vi "2_2_PatchCore_Inference(Camera).vi"() -> ()   [LabVIEW 2024]
uses:
  <vilib>/Ngene/DeepLTK Anomaly Detection Addon/DeepLTK_Anomaly_Detection_Addon/API/Controls/NN_Paths.ctl
  <vilib>/Ngene/Deep Learning Toolkit/Toolkit/NN_Data/API/NN_Dims(C,H,W).ctl
  <vilib>/Ngene/Deep Learning Toolkit/Toolkit/NN_Network/Controls/NN_Device.ctl
  subVIs/Visualizer/Controls/Display_Options.ctl
  subVIs/Visualizer/Controls/ROI_Display_Options.ctl
  subVIs/Visualizer/Controls/Heatmap_Display_Options.ctl
  subVIs/Visualizer/Controls/ColorMap.ctl
  <vilib>/Ngene/DeepLTK Anomaly Detection Addon/DeepLTK_Anomaly_Detection_Addon/API/Controls/MinMax.ctl
  subVIs/Camera/Controls/Camera_Settings.ctl
  <vilib>/vision/driver/IMAQdx.llb/IMAQdx Camera Control Mode.ctl
  <vilib>/Ngene/DeepLTK Anomaly Detection Addon/DeepLTK_Anomaly_Detection_Addon/API/Controls/NNPC_Setup.ctl
  <vilib>/Ngene/DeepLTK Anomaly Detection Addon/DeepLTK_Anomaly_Detection_Addon/API/Controls/Feature_Scorer_Params.ctl
  <vilib>/Ngene/DeepLTK Anomaly Detection Addon/DeepLTK_Anomaly_Detection_Addon/API/Controls/Gaussian_Blur.ctl
  <vilib>/vision/driver/IMAQdx.llb/IMAQdx Buffer Number Mode.ctl
  <vilib>/Ngene/DeepLTK Anomaly Detection Addon/DeepLTK_Anomaly_Detection_Addon/API/NNPC_Predict/NNPC_Predict(Single).vi
  <vilib>/Ngene/DeepLTK Anomaly Detection Addon/DeepLTK_Anomaly_Detection_Addon/DeepLTK_Anomaly_Detection_Addon.lvlib
  <vilib>/ptbypt/NI_PtbyPt.lvlib
  <vilib>/vision/driver/NI_Vision_Acquisition_Software.lvlib
  <vilib>/Ngene/Deep Learning Toolkit/Toolkit/Deep_Learning_Toolkit_by_Ngene.lvlib
panel:
  in  "Tab Control 2":enum32{"CFG", "Demo"}(tab)
  out "dT_Forward":dbl=0.5810284729999466 format="%#_3p"
  in  "Stop":bool
  out "Dims_In":T1={"C"=3, "H"=224, "W"=224}
  out "Loop Time":dbl=0.8034906005000266 format="%.2ps"
  out "Preproc. Time":dbl=0.010750834499958728 format="%.2ps"
  in  "Image_Thrshld":sgl=-1.0 format="%_5g"
  out "Pixel_Score(Max)":sgl=14.516328
  out "Img_Score":sgl=14.816199
  in  "Pixel_Thrshld":sgl=8.400001 format="%_5g"
  out "Error Count":i16
  in  "Camera_Settings":T2={"Camera_Resolution"=203, "Focus"=35, "Exposure"=5, "Gain"=50, "WhiteB."=6457} {"WhiteB." min=2000 max=7500 step=1; "Gain" max=255 step=1; "Exposure" min=0 max=9 step=1; "Focus" step=5}
  in  "Rel Margin":sgl=0.02
  in  "Camera":refnum<k21>="cam2" caption="IMAQdx Session"
  in  "Display_Options":T3={"ROI_Options"={"Color"=16711713, "Width"=4, "Drawing Mode"=enum."Frame"}, "Heatmap_Options"={"ColorMap"=enum."Jet", "Alpha"=0.4, "Heatmap Range"={"Min"=8.0, "Max"=-1.0}}, "Has GT?"=FALSE} {"Heatmap_Options"."Heatmap Range"."Min" format="%#_5g"}
  in  "Trained_Model_Paths":T8={"CFG"=path "D:/Ngene/GitHub/niconnect2025/VAD_Card_RT_v2.0_vad2.1/Models/3_Clubs_Demo_v2/NNPC_3Clubs__25_04_23__20_03_43_Fast/NNPC_3Clubs.cfg", "BIN"=path "D:/Ngene/GitHub/niconnect2025/VAD_Card_RT_v2.0_vad2.1/Models/3_Clubs_Demo_v2/NNPC_3Clubs__25_04_23__20_03_43_Fast/NNPC_3Clubs.bin"}
  in  "Device":T9
  in  "Center_Crop_Size":i32=680
  out "Prediction":bool=TRUE
  out "Device Name":string="sbRIO-9609"
  out "Inference Time":dbl=0.7674025689999553 format="%_3ps"
  out "FPS":dbl=1.3030970189520674 format="%.2f"
  out "Anomaly Detection Results":T10(plugin-control)
  # "Unsupervised \nVisual Anomaly Detection"
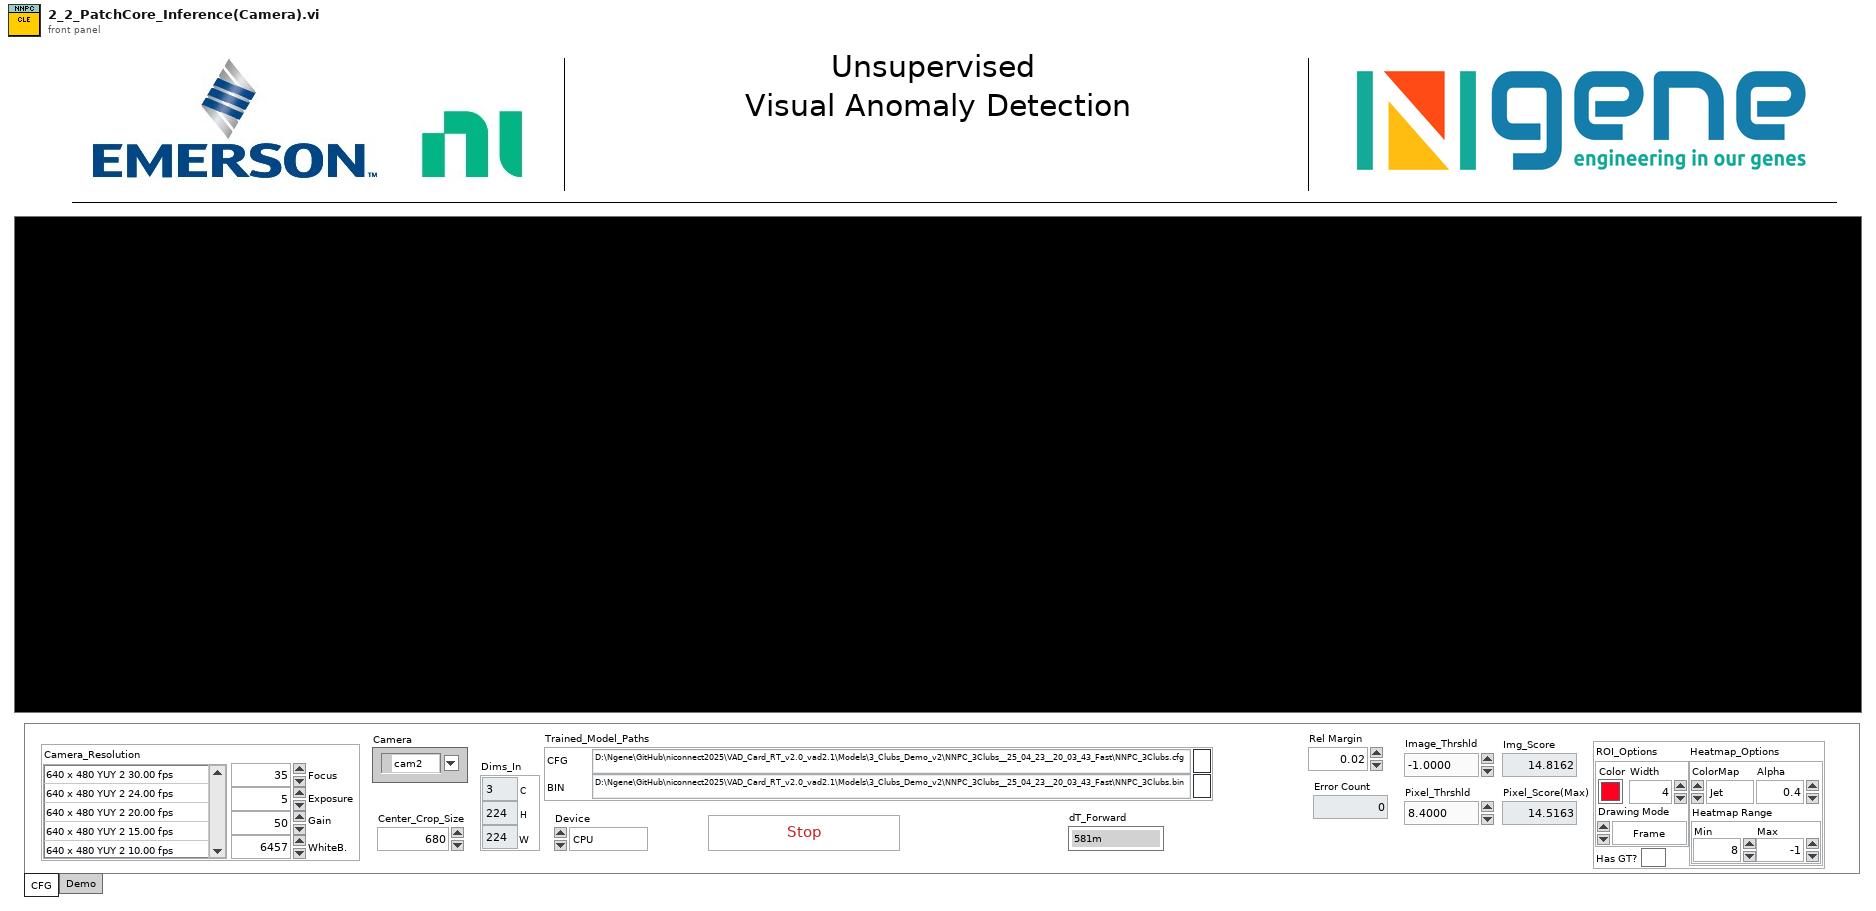
[diagram p1: front panel]
types:
  T1 = typedef "Deep_Learning_Toolkit_by_Ngene.lvlib/NN_Dims(C,H,W).ctl" = cluster{"C":i32, "H":i32, "W":i32}
  T2 = typedef "Camera_Settings.ctl" = cluster{"Camera_Resolution":i32, "Focus":u8, "Exposure":i32, "Gain":u32, "WhiteB.":i32}
  T3 = typedef "Display_Options.ctl" = cluster{"ROI_Options":T4, "Heatmap_Options":T5, "Has GT?":bool}
  T4 = typedef "ROI_Display_Options.ctl" = cluster{"Color":u32, "Width":u32, "Drawing Mode":enum16{"Frame", "Fill"}}
  T5 = typedef "Heatmap_Display_Options.ctl" = cluster{"ColorMap":T6, "Alpha":sgl, "Heatmap Range":T7}
  T6 = typedef "ColorMap.ctl" = enum16{"Jet", "Perula", "Inferno", "Plasma", "Viridis"}
  T7 = typedef "DeepLTK_Anomaly_Detection_Addon.lvlib/MinMax.ctl" = cluster{"Min":sgl, "Max":sgl}
  T8 = typedef "DeepLTK_Anomaly_Detection_Addon.lvlib/NN_Paths.ctl" = cluster{"CFG":path, "BIN":path}
  T9 = typedef "Deep_Learning_Toolkit_by_Ngene.lvlib/NN_Device.ctl" = enum16{"CPU", "GPU"}
  T10 = typedef "IMAQ Image.ctl" = refnum<image>
  T11 = typedef "Image Type" = u32
  T12 = typedef "NI_Vision_Acquisition_Software.lvlib/IMAQdx Camera Control Mode.ctl" = enum32{"Controller", "Listener"}
  T13 = typedef "DeepLTK_Anomaly_Detection_Addon.lvlib/NNPC_Setup.ctl" = cluster{"Input_Dims":T1, "mBatch":i32, "Device":T9, "GPU Id":i32}
  T14 = typedef "IMAQdx.ctl" = refnum<k21>
  T15 = typedef "DeepLTK_Anomaly_Detection_Addon.lvlib/NNPC_Evaluation_Results.ctl" = cluster{"Threshold(Image)":sgl, "Threshold(Pixel)":sgl, "Pixel_Range":cluster{"Min":sgl, "Max":sgl}}
  T16 = typedef "DeepLTK_Anomaly_Detection_Addon.lvlib/NNPC_PreProcessing_Options.ctl" = cluster{"DS_Name":string, "Input_Dims":T1, "Center Crop Size":i32, "Interpolation Type":u32, "Multi-Stage_DownSample?":bool, "Dataset_Stats":T17}
  T17 = typedef "DeepLTK_Anomaly_Detection_Addon.lvlib/NNPC_DS_Stats.ctl" = cluster{"means":T18, "stds":T18}
  T18 = typedef "DeepLTK_Anomaly_Detection_Addon.lvlib/Image_Stats_RGB.ctl" = cluster{"R":sgl, "G":sgl, "B":sgl}
  T19 = typedef "DeepLTK_Anomaly_Detection_Addon.lvlib/NNPC_Instance.ctl" = cluster{"NN out":T20, "MemBank_Data":T35, "Name":string}
  T20 = typedef "Deep_Learning_Toolkit_by_Ngene.lvlib/NN.ctl" = cluster{"Name":string, "No of Layers":i32, "mBatch":i32, "Layers":T21[], "Dimty":T22, "Dims_In":T1, "Dims_Out":T1, "Working_Dir":path, "Train?":bool, "Train_Params":T23, "LR_Update_Policy":T26, "Session Data":T28, "Ground_truth":T29, "NNg_hdls":T30, "NN_Device":T9, "GPU Id":i32, "Labels":string[], "Receptive Field":T31[], "Loss_Type":T32, "Loss_Cfg_Prms":variant, "NNG_WS":T33}
  T21 = typedef "Deep_Learning_Toolkit_by_Ngene.lvlib/NN_Layer_ref.ctl" = refnum<data-value>
  T22 = typedef "Deep_Learning_Toolkit_by_Ngene.lvlib/NN_In_Out_Dim-ty.ctl" = enum8{"In1D_Out1D", "In3D_Out1D", "In3D_Out3D", "In3D_OutBBox"}
  T23 = typedef "Deep_Learning_Toolkit_by_Ngene.lvlib/NN_Train_Params.ctl" = cluster{"Optimizer":T24, "Beta_1":sgl, "Beta_2":sgl, "Weight Decay(L1)":sgl, "Weight Decay(L2)":sgl, "Data_Sampling":T25}
  T24 = typedef "Deep_Learning_Toolkit_by_Ngene.lvlib/NN_Train_Optimizer.ctl" = enum16{"SGD", "Adam", "Adagrad", "Adadelta", "RMSProp", "Nesterov"}
  T25 = typedef "Deep_Learning_Toolkit_by_Ngene.lvlib/NN_Train_Data_Sampling.ctl" = enum16{"Random", "Sequential"}
  T26 = typedef "Deep_Learning_Toolkit_by_Ngene.lvlib/NN_LR_Policy_Cfg.ctl" = cluster{"Policy_Type":T27, "LR0":dbl, "k":sgl, "WarmUp_Policy":enum16{"Step", "Ramp"}, "WarmUp_Iter":i32, "WarmUp_Ratio":sgl}
  T27 = typedef "Deep_Learning_Toolkit_by_Ngene.lvlib/NN_LR_Policy_Type.ctl" = enum16{"Manual", "Step", "Exp", "1/t"}
  T28 = typedef "Deep_Learning_Toolkit_by_Ngene.lvlib/NN_Train_Session_Data.ctl" = cluster{"Epochs":sgl, "Tot_Iter":i32, "LR":sgl, "LR_iter":i32}
  T29 = typedef "Deep_Learning_Toolkit_by_Ngene.lvlib/NN_Ground_truth.ctl" = cluster{"Y":variant}
  T30 = typedef "Deep_Learning_Toolkit_by_Ngene.lvlib/nng_cuda_handles.ctl" = cluster{"cudnn":u64, "cublas":u64, "stream":u64, "curand":u64}
  T31 = typedef "Deep_Learning_Toolkit_by_Ngene.lvlib/NN_Dims(V,H).ctl" = cluster{"V":i32, "H":i32}
  T32 = typedef "Deep_Learning_Toolkit_by_Ngene.lvlib/NN_Loss_Type.ctl" = enum16{"None", "MSE", "CrossEntropy", "YOLO_v2", "YOLO_v4"}
  T33 = typedef "Deep_Learning_Toolkit_by_Ngene.lvlib/NNG_WS.ctl" = cluster{"NNG_WS_Mem":T34, "Max_WS_Size":i64}
  T34 = typedef "Deep_Learning_Toolkit_by_Ngene.lvlib/NNg_WS_Mem_DVR.ctl" = refnum<data-value>
  T35 = typedef "DeepLTK_Anomaly_Detection_Addon.lvlib/MemBank_and_Norm_Variants.ctl" = cluster{"MemBank":variant, "MemBank Norm":variant}
  T36 = typedef "DeepLTK_Anomaly_Detection_Addon.lvlib/Feature_Scorer_Params.ctl" = cluster{"Nearest_Neighbors":i32, "Calculate Anomaly Map":bool, "Gaussian_Blur":T37}
  T37 = typedef "DeepLTK_Anomaly_Detection_Addon.lvlib/Gaussian_Blur.ctl" = cluster{"Kernel_Size":i32, "Sigma":sgl}
  T38 = typedef "NI_Vision_Acquisition_Software.lvlib/IMAQdx Buffer Number Mode.ctl" = enum32{"Next", "Last", "Buffer Number", "Every", "Last New"}
  T39 = typedef "Anomaly_Detection_Results_Imgs.ctl" = cluster{"Image":T10, "Ground Truth":T10, "Predicted Heat Map":T10, "Predicted Mask":T10, "Segmentation":T10}
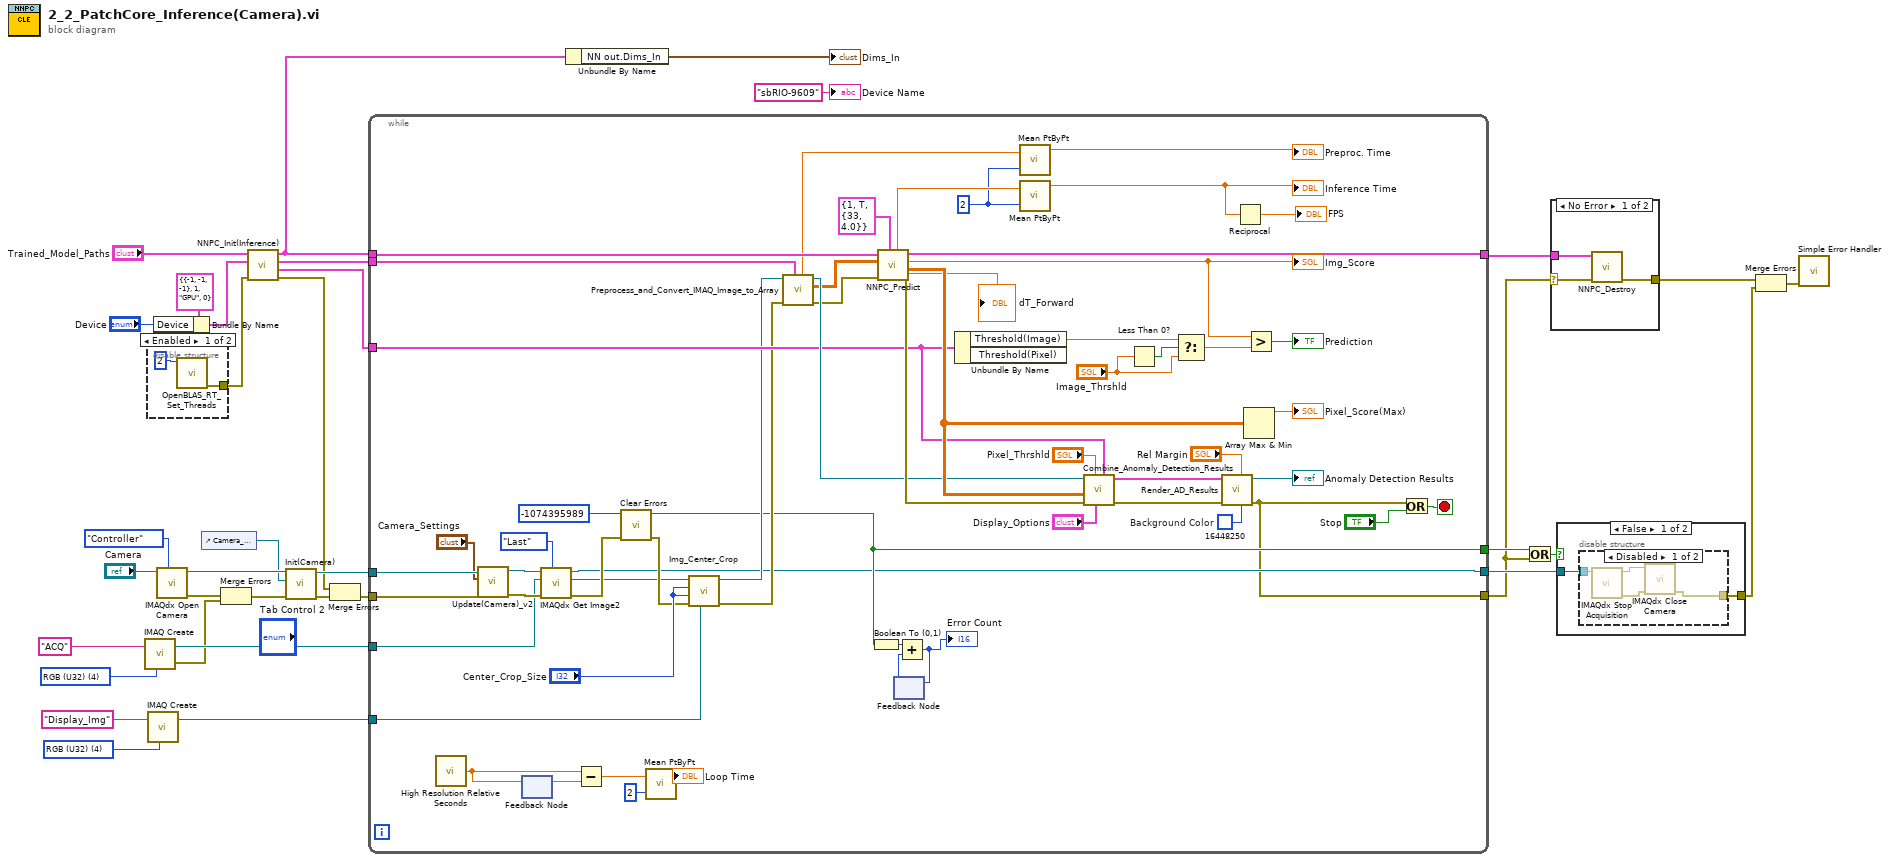
[diagram p0: block diagram]
diagram:
  w6 = T11 4 items=["Grayscale (U8)", "Grayscale (I16)", "Grayscale (SGL)", "Complex (CSG)", "RGB (U32)", "HSL (U32)", "RGB (U64)", "Grayscale (U16)"] ("Image Type")
  w19 = T11 4 items=["Grayscale (U8)", "Grayscale (I16)", "Grayscale (SGL)", "Complex (CSG)", "RGB (U32)", "HSL (U32)", "RGB (U64)", "Grayscale (U16)"] ("Image Type")
  n1 = call "IMAQ Create"("Image Name"="ACQ", "Image Type"=w19) -> ("New Image"=w14:T10, "error out"=w11:errorcluster)  [unwired: 3 in]
  n2 = disable-structure shown="Enabled" {
    disable-tunnel: [w37 _] -> w7
    frame Enabled {
      n3 = call "OpenBLAS_RT_Set_Threads.vi"("threads"=2) -> ("error out"=w37:errorcluster)  [unwired: 10 in]
    }
    frame Disabled {
    }
  }
  n4 = call "IMAQ Create"("Image Name"="Display_Img", "Image Type"=w6) -> ("New Image"=w4:T10)  [unwired: 3 in, 1 out]
  n5 = Bundle By Name(cluster=T13 {"Input_Dims"={"C"=-1, "H"=-1, "W"=-1}, "mBatch"=1, "Device"=enum."GPU", "GPU Id"=0} ("NNFE_CFG"), "Device"="Device") -> (w13:T13)
  n6 = call <vilib>:"IMAQdx Open Camera.vi"("Camera Control Mode"=IMAQdx_Camera_Control_Mode."Controller", "Session In"="Camera") -> ("error out"=w20:errorcluster, "Session Out"=w21:T14)  [unwired: 1 in, 7 out]
  n7 = control-ref of="Camera_Settings"() -> (w12:refnum<vi>)
  n8 = Merge Errors(w20, w11) -> (w17:errorcluster)
  n9 = call <vilib>:"NNPC_Init(Inference).vi"("error in"=w7, "NNPC_Setup"=w13, "NNPC_Paths"="Trained_Model_Paths") -> ("error out"=w9:errorcluster, "Evaluation_Results"=w31:T15, "PreProc_Options"=w32:T16, "NNPC_out"=w27:T19)  [unwired: 4 in, 1 out]
  n10 = call "Init(Camera).vi"("error in (no error)"=w17, "Camera_Settings_Ref"=w12, "Session in"=w21) -> ("error out"=w16:errorcluster, "Session out"=w15:T14)  [unwired: 7 in]
  n11 = Merge Errors(w9, w16) -> (w10:errorcluster)
  n12 = while {
    tunnel: w27 -> [w86]
    tunnel: [w81] -> w35
    tunnel: w32 -> [w73]
    tunnel: w31 -> [w68]
    tunnel: [w43] -> w30
    tunnel: [w42] -> w1
    tunnel: w10 -> [w61]
    tunnel: w15 -> [w64]
    tunnel: w14 -> [w60]
    tunnel: w4 -> [w50]
    tunnel: [w47] -> w3
    stop <- w80 stop-if-true
    w41 = 2 ("sample length")
    w79 = u32 16448250  # Background Color
    n13 = call <vilib>:"High Resolution Relative Seconds.vi"() -> ("relative seconds"=w75:dbl)
    n14 = call "Update(Camera)_v2.vi"("error in (no error)"=w61, "Camera_Settings"="Camera_Settings", "Session in"=w64) -> ("error out"=w63:errorcluster, "Session out"=w62:T14)  [unwired: 7 in]
    n15 = feedback #1() -> (w76:dbl)  [unwired: 1 in]
    n16 = feedback-in #1(w75) -> ()
    n17 = call <vilib>:"IMAQdx Get Image2.vi"("Buffer Number Mode (Next)"=IMAQdx_Buffer_Number_Mode."Last", "error in"=w63, "Image In"=w60, "Session In"=w62) -> ("error out"=w52:errorcluster, "Image Out"=w51:T10, "Session Out"=w43:T14)  [unwired: 4 in, 1 out]
    n18 = Subtract(x=w75, y=w76) -> (x-y=w74:dbl)
    n19 = call <vilib>:"Clear Errors.vi"("error in (no error)"=w52, "specific error code to clear (0: all)"=-1074395989) -> ("error out"=w54:errorcluster, "specific error cleared?"=w47:bool)  [unwired: 4 in]
    n20 = call <vilib>:"Mean PtByPt.vi"("x"=w74, "sample length"=2) -> ("mean"=→"Loop Time":dbl)  [unwired: 2 in, 1 out]
    n21 = call "Img_Center_Crop.vi"("Image Dst"=w50, "error in (no error)"=w54, "height"="Center_Crop_Size", "width"="Center_Crop_Size", "Image In"=w51) -> ("error out"=w56:errorcluster, "Image Out"=w58:T10)  [unwired: 5 in]
    n22 = call "Preprocess_and_Convert_IMAQ_Image_to_Array.vi"("PreProcessing_Options"=w73, "error in (no error)"=w56, "Imaq Image In"=w58) -> ("error out"=w69:errorcluster, "Norm_Img_Out"=w55:sgl[][][], "Imaq Image Out"=w70:T10, "dT_Preprocessing"=w71:dbl)  [unwired: 5 in]
    n23 = Boolean To (0,1)(Boolean=w47) -> (0, 1=w46:i16)
    n24 = call-poly <vilib>:"NNPC_Predict.vi"("Feature_Scorer_Params"=T36 {"Nearest_Neighbors"=1, "Calculate Anomaly Map"=TRUE, "Gaussian_Blur"={"Kernel_Size"=33, "Sigma"=4.0}}, "error in"=w69, "Image_in"=w55, "NNPC_in"=w86) -> ("error out"=w96:errorcluster, "Anomaly_Map"=w85:sgl[][], "Pred_Score"=w84:sgl, "NNPC_out"=w81:T19, "dT_Forward"=→"dT_Forward":dbl, "dT_Predict"=w78:dbl)  [unwired: 2 in]
    "Img_Score" <- w84
    n25 = feedback #2() -> (w48:i16)  [unwired: 1 in]
    n26 = Add(x=w46, y=w48) -> (x+y=w45:i16)
    "Error Count" <- w45
    n27 = feedback-in #2(w45) -> ()
    n28 = Unbundle By Name(w68) -> ("Threshold(Image)"=w77:sgl)  [unwired: 1 out]
    n29 = call <vilib>:"Mean PtByPt.vi"("x"=w71, "sample length"=w41) -> ("mean"=→"Preproc. Time":dbl)  [unwired: 2 in, 1 out]
    n30 = call <vilib>:"Mean PtByPt.vi"("x"=w78, "sample length"=w41) -> ("mean"=w40:dbl)  [unwired: 2 in, 1 out]
    "Inference Time" <- w40
    n31 = call "Combine_Anomaly_Detection_Results.vi"("Evaluation_Results"=w68, "Display_Options"="Display_Options", "Pixel Anomaly Thrshld"="Pixel_Thrshld", "error in"=w96, "Anomaly Map"=w85, "Orig Image In"=w70) -> ("error out"=w95:errorcluster, "Anomaly Detection Rresults"=w94:T39)  [unwired: 3 in, 1 out]
    n32 = Less Than 0?(x="Image_Thrshld") -> (x < 0?=w90:bool)
    n33 = Select(t=w77, s=w90, f="Image_Thrshld") -> (s? t:f=w88:sgl)
    n34 = call "Render_AD_Results.vi"("Background Color"=w79, "Rel._Margin"="Rel Margin", "error in"=w95, "Anomaly Detection Rresults"=w94) -> ("error out"=w42:errorcluster, "Anomaly Detection Results"=→"Anomaly Detection Results":T10)  [unwired: 6 in]
    n35 = Reciprocal(x=w40) -> (1/x=→"FPS":dbl)
    n36 = Array Max & Min(array=w85) -> (max value=→"Pixel_Score(Max)":sgl)  [unwired: 3 out]
    n37 = Greater?(x=w84, y=w88) -> (0:→"Prediction":bool)
    n38 = Or(x=w42, y="Stop") -> (x .or. y?=w80:bool)
  }
  n39 = Unbundle By Name(w27) -> ("NN out.Dims_In"=→"Dims_In":T1)
  n40 = Or(x=w3, y=w1) -> (x .or. y?=w2:bool)
  n41 = case shown="No Error" w1 {
    selector: w1 -> [w97 w100]
    tunnel: w35 -> [w99 _]
    tunnel: [w98 w100] -> w34
    frame No Error {
      n42 = call <vilib>:"NNPC_Destroy.vi"("error in"=w97, "NNPC_in"=w99) -> ("error out"=w98:errorcluster)  [unwired: 9 in]
    }
    frame Error {
    }
  }
  n43 = case shown="False" w2 {
    tunnel: w30 -> [w102 _]
    tunnel: [w101 _] -> w28
    frame False {
      n44 = disable-structure shown="Disabled" {
        disable-tunnel: w102 -> [w106 _]
        disable-tunnel: [w103 _] -> w101
        frame Disabled {
          n45 = call <vilib>:"IMAQdx Stop Acquisition.vi"("Session In"=w106) -> ("error out"=w104:errorcluster, "Session Out"=w105:T14)  [unwired: 9 in]
          n46 = call <vilib>:"IMAQdx Close Camera.vi"("error in"=w104, "Session In"=w105) -> ("error out"=w103:errorcluster)  [unwired: 9 in]
        }
        frame Enabled {
        }
      }
    }
    frame True {
    }
  }
  n47 = Merge Errors(w34, w28) -> (w29:errorcluster)
  n48 = call <vilib>:"Simple Error Handler.vi"("error in (no error)"=w29) -> ()  [unwired: 4 in, 5 out]
  "Device Name" <- "sbRIO-9609" ("Device Name")
